vi "geve-populate_log.vi"(8 "error in (no error)":errorcluster, 11 "String in":string) -> (0 "error out":errorcluster, 3 "log out":string)   [LabVIEW 2018]
doc: "populate log."
uses:
  ee074700-d42d-4511-8373-8bddbf80cc80.vi
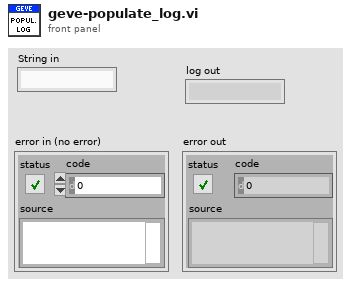
[diagram p1: front panel]
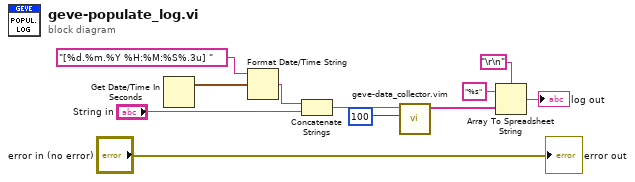
[diagram p0: block diagram]
diagram:
  n1 = Get Date/Time In Seconds() -> (seconds since 1Jan1904=w7:timestamp)
  n2 = Format Date/Time String(time format string (%c)="[%d.%m.%Y %H:%M:%S%.3u] ", seconds (now)=w7) -> (date/time string=w9:string)  [unwired: 1 in]
  n3 = Concatenate Strings(w9, "String in") -> (w10:string)
  n4 = call "geve-data_collector.vim"("Max Values"=100, "Time Stamp"=w10) -> ("Time Stamp Array"=w5:string[])  [unwired: 9 in]
  n5 = Array To Spreadsheet String(delimiter (Tab)="\r\n", array=w5, 3:"%s" ("format string")) -> (spreadsheet string=→"log out":string)
  "error out" <- "error in (no error)"
